vi "告警码字段定义.vi"(10 "首次调用？":bool, 11 "告警代码":u16) -> (3 "data":T1)   [LabVIEW 2016, in "斯坦道CODMn新电路板.lvlib"]
uses:
  Alarm interface/Alarm interface.lvlib
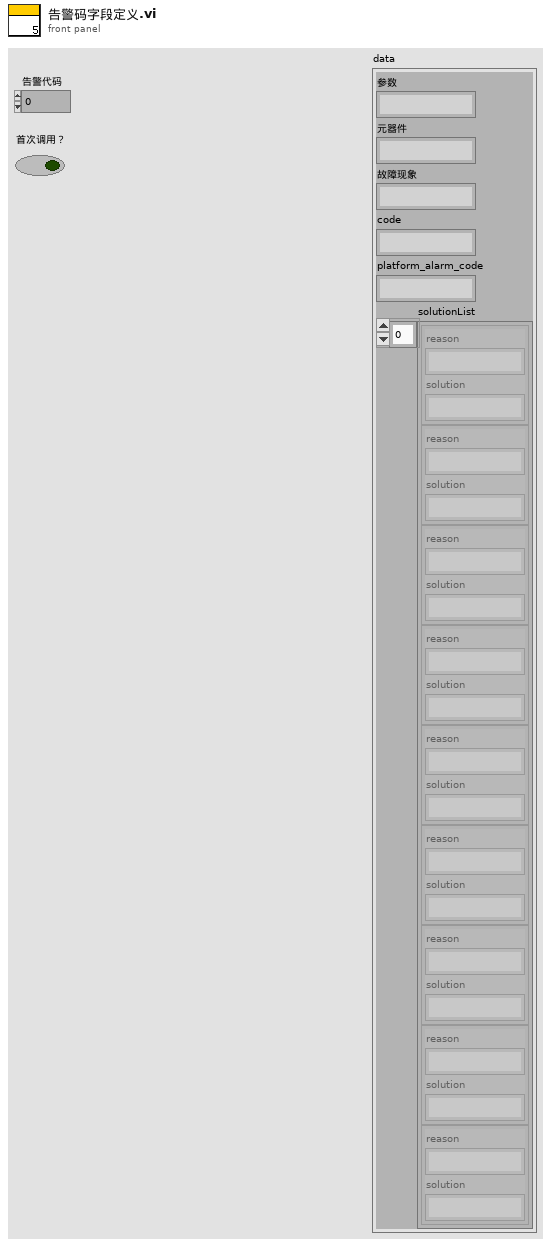
[diagram p1: front panel]
types:
  T1 = typedef "Alarm interface.lvlib/报警短信语音交互.ctl" = cluster{"参数":string, "元器件":string, "故障现象":string, "code":string, "platform_alarm_code":string, "solutionList":cluster{"reason":string, "solution":string}[]}
  T2 = cluster{"componentParent":string, "equipVersion":string, string}
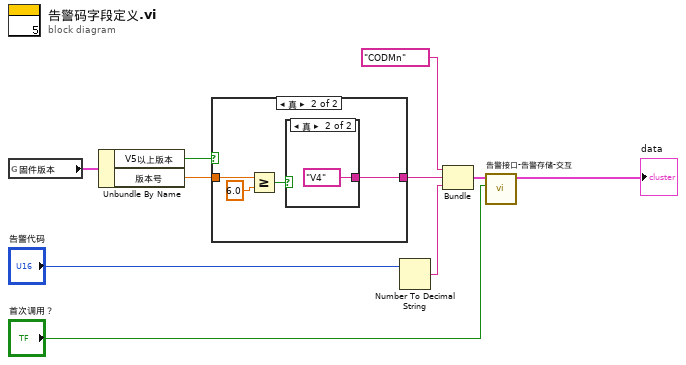
[diagram p0: block diagram]
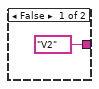
[diagram p2: hidden frame]
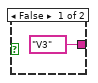
[diagram p3: hidden frame]
diagram:
  n1 = global read "VARCODMn全局变量.vi" "固件版本"() -> (w3:cluster{"V5以上版本":bool, "版本号":dbl})
  n2 = Unbundle By Name(w3) -> ("V5以上版本"=w2:bool, "版本号"=w1:dbl)
  n3 = case shown="真" w2 {
    tunnel: ["V2" ("equipVersion") w15] -> w8
    tunnel: w1 -> [_ w13]
    frame False {
    }
    frame True {
      n4 = Greater Or Equal?(x=w13, y=6.0) -> (x >= y?=w12:bool)
      n5 = case shown="真" w12 {
        tunnel: ["V3" ("equipVersion") "V4" ("equipVersion")] -> w15
        frame False {
        }
        frame True {
        }
      }
    }
  }
  n6 = Number To Decimal String(number="告警代码") -> (decimal integer string=w9:string)  [unwired: 1 in]
  n7 = Bundle("componentParent"="CODMn", "equipVersion"=w8, w9) -> (w7:T2)  [unwired: 1 in]
  n8 = call "告警接口-告警存储-交互.vi"("首次调用？"="首次调用？", "筛选输入"=w7) -> ("data"=→"data":T1)  [unwired: 8 in, 1 out]
